vi "CTRE_Phoenix_MotorControl_BufferedTrajectoryPointStream_WriteOne.vi"(8 "error in":errorcluster, 10 "Trajectory Point":T2, 11 "BufferedTrajectoryPointStream_DevRef":T1) -> (0 "error out":errorcluster, 3 "BufferedTrajectoryPointStream_DevRef":T1)   [LabVIEW 2020]
doc: "Push a single trajectory point into the Buffered Stream"
uses:
  <vilib>/Rock Robotics/WPI/ThirdParty/Phoenix-LabVIEW/Motor Controller/Controls/CTRE_Phoenix_MotorControl_MotionProfileTrajectoryPoint.ctl
  <vilib>/Rock Robotics/WPI/ThirdParty/Phoenix-LabVIEW/Motor Controller/Controls/CTRE_Phoenix_MotorControl_BufferedTrajectoryPointStream_DeviceRef.ctl
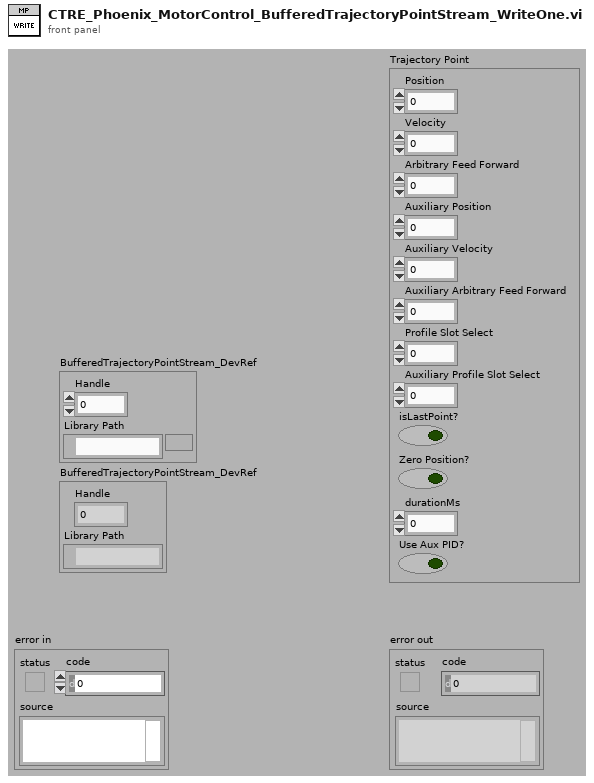
[diagram p1: front panel]
types:
  T1 = typedef "CTRE_Phoenix_MotorControl_BufferedTrajectoryPointStream_DeviceRef.ctl" = cluster{"Handle":u64, "Library Path":path}
  T2 = typedef "CTRE_Phoenix_MotorControl_MotionProfileTrajectoryPoint.ctl" = cluster{"Position":dbl, "Velocity":dbl, "Arbitrary Feed Forward":dbl, "Auxiliary Position":dbl, "Auxiliary Velocity":dbl, "Auxiliary Arbitrary Feed Forward":dbl, "Profile Slot Select":i32, "Auxiliary Profile Slot Select":i32, "isLastPoint?":bool, "Zero Position?":bool, "durationMs":u32, "Use Aux PID?":bool}
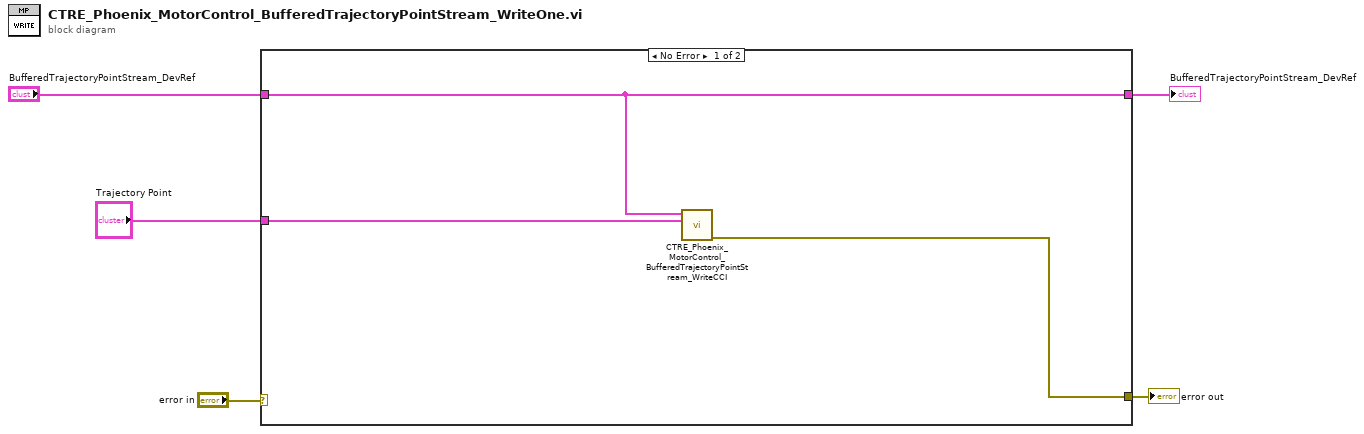
[diagram p0: block diagram]
diagram:
  n1 = case shown="No Error" "error in" {
    selector: "error in" -> [_ w10]
    tunnel: [w6 w10] -> w5
    tunnel: [w7 w9] -> w2
    tunnel: "BufferedTrajectoryPointStream_DevRef" -> [w7 w9]
    tunnel: "Trajectory Point" -> [w8 _]
    frame No Error {
      n2 = call <vilib>:"CTRE_Phoenix_MotorControl_BufferedTrajectoryPointStream_WriteCCI.vi"("Trajectory Point"=w8, "BufferedTrajectoryPointStream_DevRef"=w7) -> ("error out"=w6:errorcluster)  [unwired: 8 in, 1 out]
    }
    frame Error {
    }
  }
  "error out" <- w5
  "BufferedTrajectoryPointStream_DevRef" <- w2
